vi "Set File Permissions V2.vi"(0 "PDF Report IN":refnum<class "PDF Report Class.lvclass">, 7 "Permissions":T1={"User Password"="", "Owner Password"="", "Printing"=enum."Allow Printing", "Allow Modify Contents"=FALSE, "Allow Copy"=FALSE, "Allow Modify Annotations"=TRUE, "Allow Fill In "=TRUE, "Allow Screen Readers"=FALSE, "Allow Assembly"=FALSE}, 11 "error in (no error)":errorcluster) -> (4 "PDF Report OUT":refnum<class "PDF Report Class.lvclass">, 15 "error out":errorcluster)   [LabVIEW 2019, in "Exaprom PDF.lvlib"]
doc: "Version 2.0\nDeveloped by Jean-Marc Simard\nCopyright © 2012, Exaprom Inc.\nAll rights reserved.\nLicense: BSD\n\nWith iTextSharp 4.1.6 (http://itextsharp.sourceforge.net)\nunder Mozilla Public License Version 1.1\n(http://www.mozilla.org/MPL/MPL-1.1.html)"
uses:
  LV Class/PDF Report Class/PDF Report Class.lvclass
  Controls/Initialization Controls/File Permission Parameters.ctl
  C:/work/niobrara_lv/labview pdf writer fixing/DLL/itextsharp.dll
  DLL/itextsharp.dll
  Exaprom PDF.lvlib
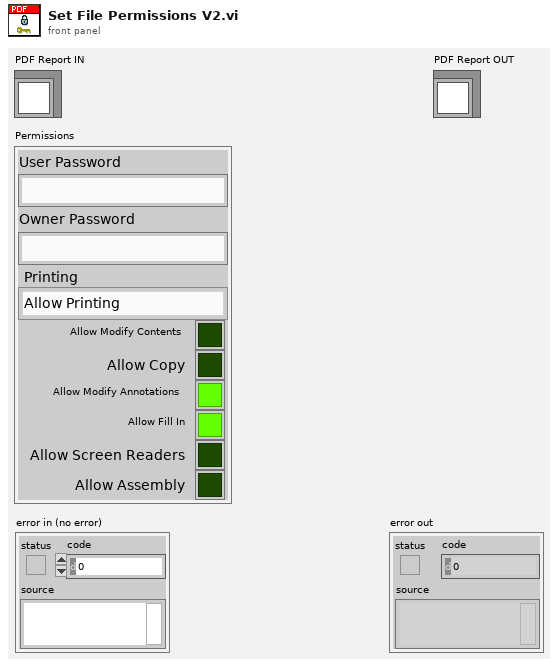
[diagram p1: front panel]
types:
  T1 = typedef "Exaprom PDF.lvlib/File Permission Parameters.ctl" = cluster{"User Password":string, "Owner Password":string, "Printing":enum16{"Allow Printing", "Allow Degraded Printing", "Don't Allow Printing"}, "Allow Modify Contents":bool, "Allow Copy":bool, "Allow Modify Annotations":bool, "Allow Fill In ":bool, "Allow Screen Readers":bool, "Allow Assembly":bool}
  T2 = cluster{"AllowAssembly":i32, "AllowCopy":i32, "AllowDegradedPrinting":i32, "AllowFillIn":i32, "AllowModifyAnnotations":i32, "AllowModifyContents":i32, "AllowPrinting":i32, "AllowScreenReaders":i32}
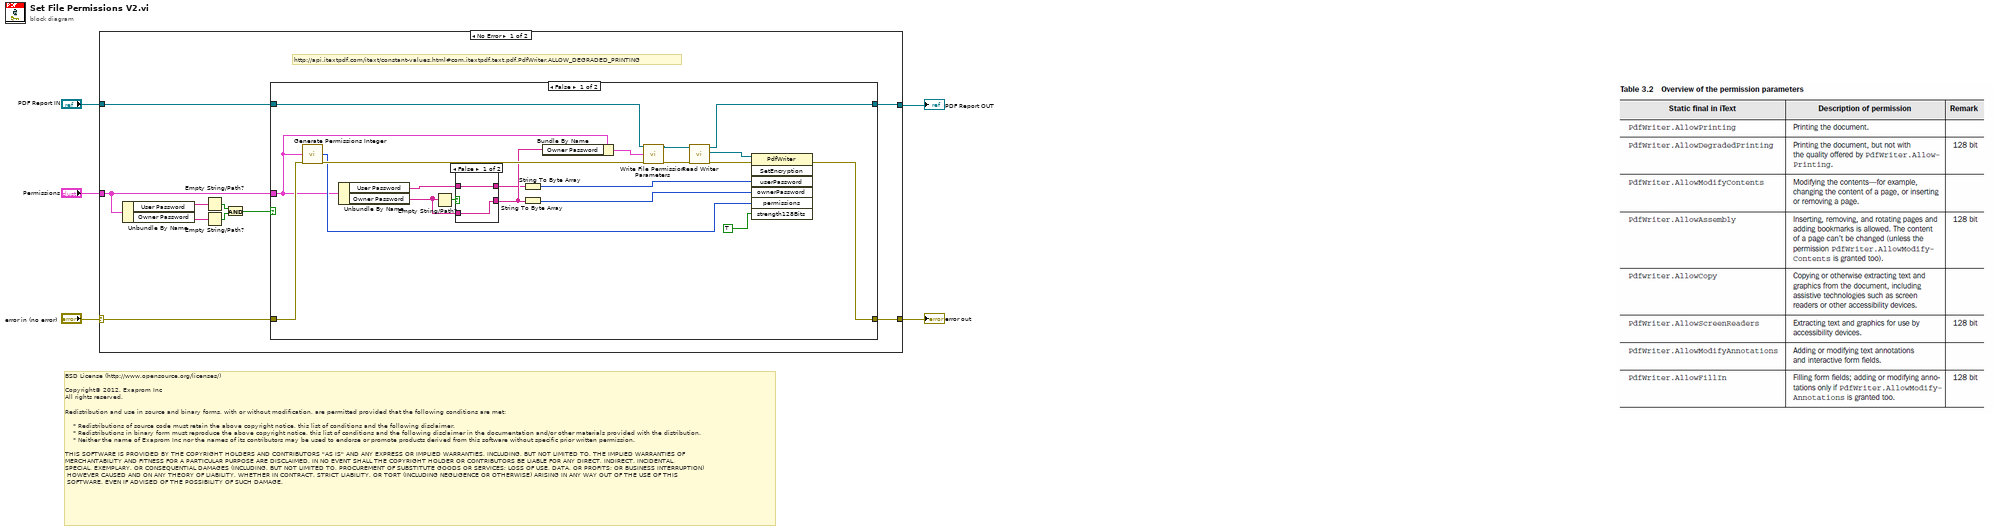
[diagram p0: block diagram]
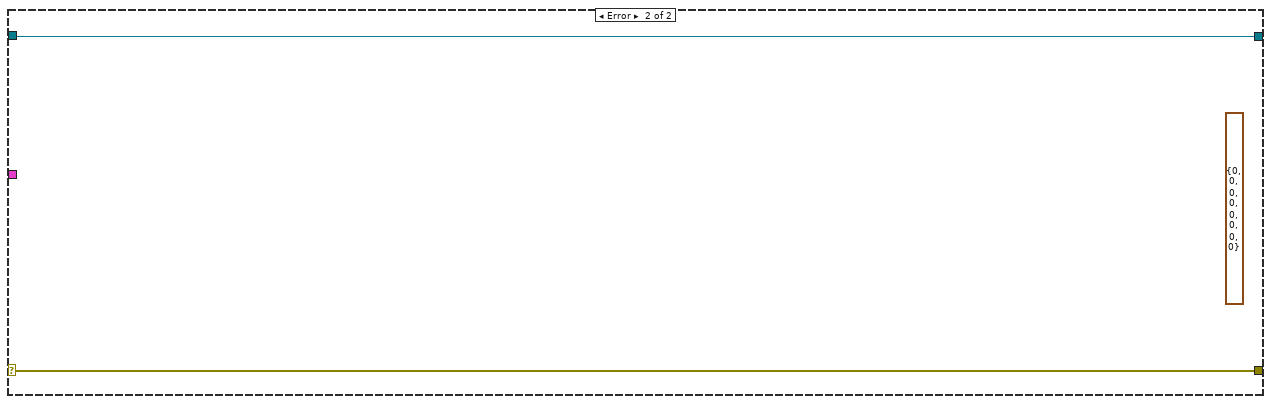
[diagram p4: hidden frame]
diagram:
  # "BSD License (http://www.opensource.org/licenses/)\n\nCopyright© 2012, Exaprom Inc\nAll rights reserved.\n\nRedistribution and use in source and binary forms, with or without modification, are permitted provided that the following conditions are met:\n\n    * Redistributions of source code must retain the above copyright notice, this list of conditions and the following disclaimer.\n    * Redistributions in binary form must reproduce the above copyright notice, this list of conditions and the following disclaimer in the documentation and/or other materials provided with the distribution.\n    * Neither the name of Exaprom Inc nor the names of its contributors may be used to endorse or promote products derived from this software without specific prior written permission.\n\nTHIS SOFTWARE IS PROVIDED BY THE COPYRIGHT HOLDERS AND CONTRIBUTORS \"AS IS\" AND ANY EXPRESS OR IMPLIED WARRANTIES, INCLUDING, BUT NOT LIMITED TO, THE IMPLIED WARRANTIES OF \nMERCHANTABILITY AND FITNESS FOR A PARTICULAR PURPOSE ARE DISCLAIMED. IN NO EVENT SHALL THE COPYRIGHT HOLDER OR CONTRIBUTORS BE LIABLE FOR ANY DIRECT, INDIRECT, INCIDENTAL,\nSPECIAL, EXEMPLARY, OR CONSEQUENTIAL DAMAGES (INCLUDING, BUT NOT LIMITED TO, PROCUREMENT OF SUBSTITUTE GOODS OR SERVICES; LOSS OF USE, DATA, OR PROFITS; OR BUSINESS INTERRUPTION)\n HOWEVER CAUSED AND ON ANY THEORY OF LIABILITY, WHETHER IN CONTRACT, STRICT LIABILITY, OR TORT (INCLUDING NEGLIGENCE OR OTHERWISE) ARISING IN ANY WAY OUT OF THE USE OF THIS\n SOFTWARE, EVEN IF ADVISED OF THE POSSIBILITY OF SUCH DAMAGE."
  n1 = case shown="No Error" "error in (no error)" {
    selector: "error in (no error)" -> [w15 w42]
    tunnel: "PDF Report IN" -> [w14 w41]
    tunnel: [w12 w41] -> w4
    tunnel: [w13 w42] -> w3
    tunnel: "Permissions" -> [w11 _]
    frame No Error {
      # "http://api.itextpdf.com/itext/constant-values.html#com.itextpdf.text.pdf.PdfWriter.ALLOW_DEGRADED_PRINTING"
      n2 = Unbundle By Name(w11) -> ("User Password"=w10:string, "Owner Password"=w9:string)
      n3 = Empty String/Path?(string/path=w10) -> (empty?=w8:bool)
      n4 = Empty String/Path?(string/path=w9) -> (empty?=w6:bool)
      n5 = And(x=w8, y=w6) -> (x .and. y?=w7:bool)
      n6 = case shown="False" w7 {
        tunnel: w15 -> [w35 w40]
        tunnel: w14 -> [w26 w39]
        tunnel: [w31 w40] -> w13
        tunnel: w11 -> [w21 _]
        tunnel: [w28 w39] -> w12
        frame False {
          n7 = call "Generate Permissions Integer.vi"("Permissions"=w21, "error in (no error)"=w35) -> ("Permissions"=w22:i32, "error out"=w30:errorcluster)  [unwired: 12 out]
          n8 = Unbundle By Name(w21) -> ("User Password"=w16:string, "Owner Password"=w24:string)
          n9 = Empty String/Path?(string/path=w24) -> (empty?=w33:bool)
          n10 = case shown="False" w33 {
            tunnel: [w37 w38] -> w18
            tunnel: w24 -> [w37 _]
            tunnel: [w36 w38] -> w17
            tunnel: w16 -> [w36 w38]
            frame False {
            }
            frame True {
            }
          }
          n11 = String To Byte Array(string=w17) -> (unsigned byte array=w34:u8[])
          n12 = String To Byte Array(string=w18) -> (unsigned byte array=w23:u8[])
          n13 = Bundle By Name(cluster=w21, "Owner Password"=w18) -> (w20:T1)
          n14 = call-dynamic "Write File Permission Parameters.vi"("PDF Report Class in"=w26, "File Permission Parameters"=w20, "error in (no error)"=w30) -> ("PDF Report Class out"=w25:refnum<class "PDF Report Class.lvclass">, "error out"=w27:errorcluster)  [unwired: 11 in]
          n15 = call-dynamic "Read Writer.vi"("error in (no error)"=w27, "PDF Report Class in"=w25) -> ("error out"=w29:errorcluster, "Writer"=w19:refnum<k24>, "PDF Report Class out"=w28:refnum<class "PDF Report Class.lvclass">)  [unwired: 7 in]
          n16 = invoke class="PdfWriter" method="SetEncryption"(reference=w19, error in=w29, "userPassword"=w34, "ownerPassword"=w23, "permissions"=w22, "strength128Bits"=TRUE) -> (error out=w31:errorcluster)  [unwired: 1 in, 6 out]
        }
        frame True {
        }
      }
    }
    frame Error {
      (unwired) T2 {"AllowAssembly"=0, "AllowCopy"=0, "AllowDegradedPrinting"=0, "AllowFillIn"=0, "AllowModifyAnnotations"=0, "AllowModifyContents"=0, "AllowPrinting"=0, "AllowScreenReaders"=0}
    }
  }
  "PDF Report OUT" <- w4
  "error out" <- w3
